vi "Read Tactics.vi"(8 "error in (no error)":errorcluster, 11 "PrimaryAttackerRole_v2 in":refnum<class "PrimaryAttackerRole_v2.lvclass">) -> (0 "error out":errorcluster, 2 "Tactics":T1, 3 "PrimaryAttackerRole_v2 out":refnum<class "PrimaryAttackerRole_v2.lvclass">)   [LabVIEW 2023, in "PrimaryAttackerRole_v2.lvclass"]
uses:
  PrimaryAttackerRole_v2.lvclass
  Tactics/InterceptBallTactic_v2_class/InterceptBallTactic_v2.lvclass
  PrimaryAttackerRole_v2.lvclass/PrimaryAttackerRole_v2.ctl
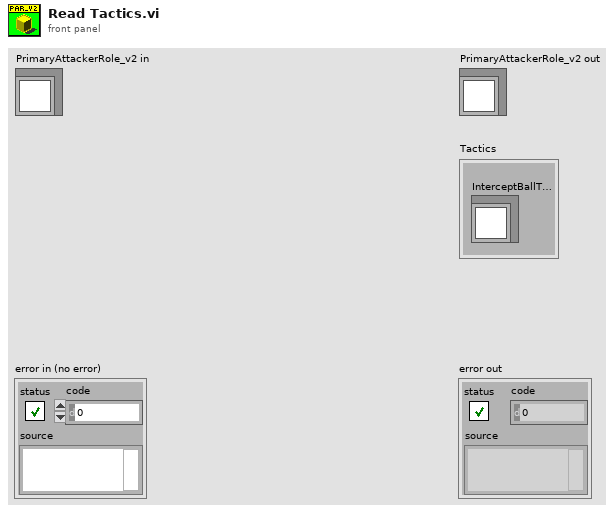
[diagram p1: front panel]
types:
  T1 = cluster{"InterceptBallTactic_v2":refnum<class "InterceptBallTactic_v2.lvclass">}
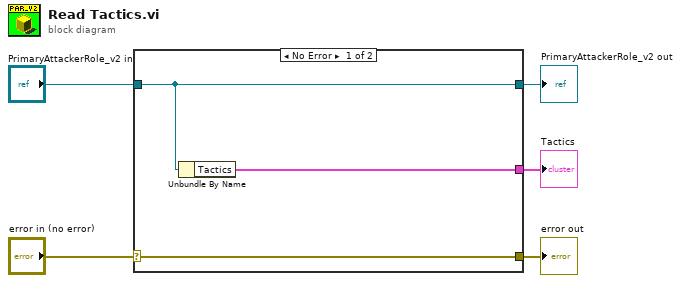
[diagram p0: block diagram]
diagram:
  n1 = case shown="No Error" "error in (no error)" {
    selector: "error in (no error)" -> [w8 w9]
    tunnel: [w8 w9] -> w4
    tunnel: [w7 w10] -> w2
    tunnel: "PrimaryAttackerRole_v2 in" -> [w7 w10]
    tunnel: [w6 _] -> w1
    frame No Error {
      n2 = Unbundle By Name(w7) -> ("Tactics"=w6:T1)
    }
    frame Error {
    }
  }
  "error out" <- w4
  "PrimaryAttackerRole_v2 out" <- w2
  "Tactics" <- w1
